vi "4 ch resonance scanner acquisition (FPGA) fixed pix clock.vi"() -> ()   [LabVIEW 2012]
uses:
  <vilib>/eio/EIONode/EIONode.xnode
  <vilib>/rvi/eio/common/nirviEmuTemplateMethod_errors.vi
  <vilib>/rvi/DataTransferAndStorage/Container/XNode/niFpgaContainer.xnode
  <vilib>/rvi/interface/RandomDataEmulation/nirviRandomDataFpgaReadWriteTemplate.vi
  <vilib>/platform/TimedLoop/XDataNode/XDataNode.xnode
  <vilib>/Platform/TimedLoop/XDataNode/nitl_modes.ctl
  <vilib>/Platform/TimedLoop/XDataNode/XDNodeRunTimeDep.lvlib
  <vilib>/Platform/TimedLoop/XDataNode/wakeup.ctl
  <vilib>/Platform/TimedLoop/XDataNode/timing_clust.ctl
panel:
  in  "lines at once":i16=4999
  in  "dwell time in ticks":i32
  in  "samples per half period":i16=4999
  in  "Start Delay (Ticks)":i16 caption="Start delay (Ticks)"
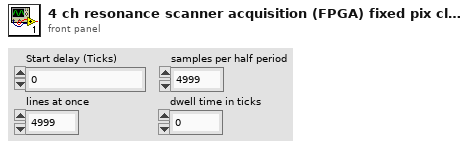
[diagram p1: front panel]
types:
  T1 = cluster{"IO Module\\AI A0":i32, "IO Module\\AI A1":i32, "IO Module\\AI A1 2":i32, "IO Module\\AI A1 3":i32}
  T2 = typedef "XDNodeRunTimeDep.lvlib/timing_clust.ctl" = cluster{"Expected End [f-1]":u64, "Actual End [f-1]":u64, "Finished Late? [f-1]":bool, "Expected End [i-1]":u64, "Actual End [i-1]":u64, "Finished Late? [i-1]":bool, "Expected Start [i]":u64, "Actual Start [i]":u64, "Expected Start [f]":u64, "Actual Start [f]":u64, "Source Name":string, "Structure Name":string, "Period":i64, "Deadline":i64, "Offset":i64, "Start":i64, "Priority":i32, "Timeout":i32, "Mode":T3, "Wakeup Reason":T4, "Error":errorcluster, "Source Type":string, "Secondary Source Type":string, "Global End Time":u64, "Global Start Time":u64, "Frame Duration":u64, "Iteration Duration":u64, "Assigned CPU":i32, "I/O Scan Engine Mode":u32}
  T3 = typedef "XDNodeRunTimeDep.lvlib/nitl_modes.ctl" = enum32{"No Change", "Process missed periods, maintain original phase", "Discard missed periods, maintain original phase", "Process missed periods, ignore original phase", "Discard missed periods, ignore original phase"}
  T4 = typedef "XDNodeRunTimeDep.lvlib/wakeup.ctl" = enum32{"Normal", "Aborted", "Asynchronous wakeup", "Timing source error", "Timed loop error", "Timeout"}
  T5 = cluster{"IO Module\\AI A0":void, "IO Module\\AI A1":void, "IO Module\\AI A2":void, "IO Module\\AI A3":void}
  T6 = cluster{"IO Module\\AI A0":i32, "IO Module\\AI A1":i32, "IO Module\\AI A2":i32, "IO Module\\AI A3":i32}
  T7 = cluster{"IO Module\\AI A0":i32, "IO Module\\AI A1":i32, i32, i32}
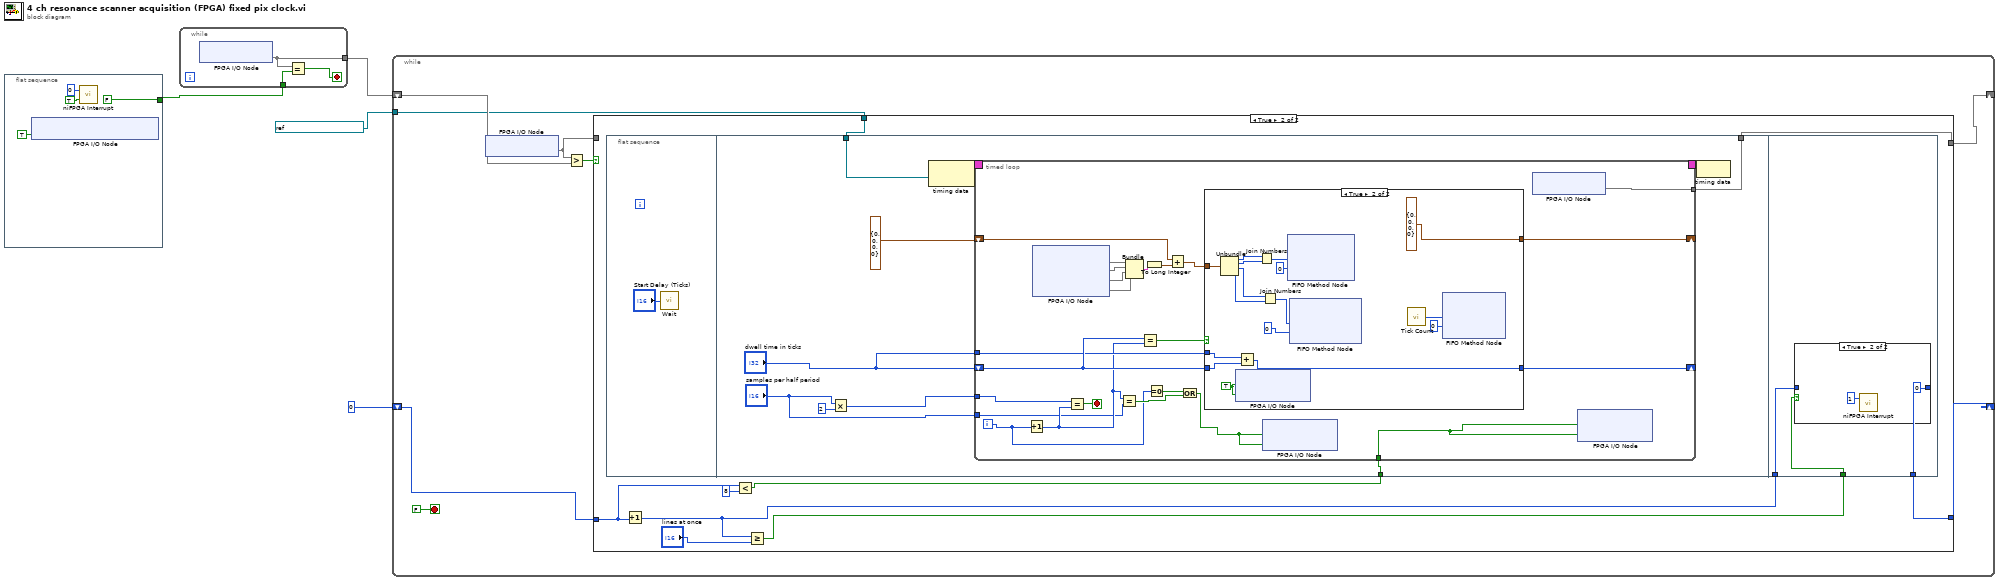
[diagram p0: block diagram]
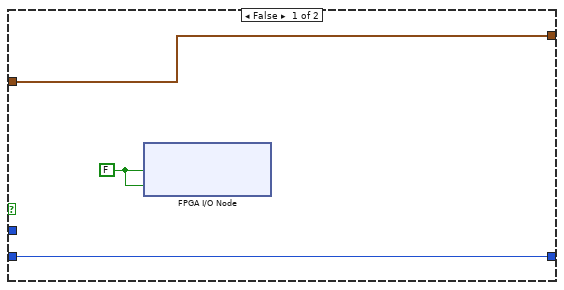
[diagram p3: hidden frame]
diagram:
  n1 = flat-sequence {
    tunnel: [FALSE ("IO Module\\DI 0")] -> w2
    frame #0 {
      n2 = xnode "FPGA I/O Node"("IO Module\\Digital Output Enable"=TRUE ("IO Module\\Digital Output Enable")) -> ()  [unwired: 1 in, 1 out]
      n3 = call <vilib>:"niFPGA Interrupt.vi"("Wait Until Cleared (F)"=TRUE, "IRQ Number (0)"=u8 0) -> ()  [unwired: 1 in]
    }
  }
  n4 = while {
    tunnel: w2 -> [w11]
    tunnel: [w9] -> w1
    stop <- w10 stop-if-true
    n5 = xnode "FPGA I/O Node"() -> ("IO Module\\DI 0"=w9)  [unwired: 1 in, 1 out]
    n6 = Equal?(x=w9, y=w11) -> (x = y?=w10:bool)
  }
  n7 = while {
    shift-right: [w18] -> _
    shift-left: w1 -> [w19]
    shift-right: [w16] -> _
    shift-left: i16 0 ("IRQ Number (0)") -> [w15]
    tunnel: refnum<k21> "40 MHz Onboard Clock" ("Source Name") -> [w13]
    stop <- FALSE stop-if-true
    n8 = xnode "FPGA I/O Node"() -> ("IO Module\\DI 0"=w12)  [unwired: 1 in, 1 out]
    n9 = Greater?(x=w12, y=w19) -> (0:w14:bool)
    n10 = case shown="True" w14 {
      tunnel: [w20 w22] -> w18
      tunnel: w15 -> [w21 w24]
      tunnel: [w21 w28] -> w16
      tunnel: w13 -> [_ w27]
      tunnel: w12 -> [w20 _]
      frame False {
      }
      frame True {
        n11 = flat-sequence {
          tunnel: w27 -> [w37]
          tunnel: w26 -> [w33]
          tunnel: [w32] -> w22
          tunnel: w30 -> [w92]
          tunnel: w29 -> [w91]
          tunnel: [w90] -> w28
          frame #0 {
            n12 = call "Wait"("Count(Ticks)"="Start Delay (Ticks)") -> ()  [unwired: 1 out]
          }
          frame #1 {
            n13 = Multiply(x="samples per half period", y=i16 2) -> (x*y=w35:i16)
            n14 = node-c288(w37) -> (w39:T2)
            n15 = timed-loop {
              tunnel: w35 -> [w63]
              shift-right: [w54] -> _
              shift-left: T1 {"IO Module\\AI A0"=0, "IO Module\\AI A1"=0, "IO Module\\AI A1 2"=0, "IO Module\\AI A1 3"=0} ("x+y") -> [w59]
              shift-right: [w57] -> _
              shift-left: "dwell time in ticks" -> [w53]
              tunnel: "dwell time in ticks" -> [w52]
              timing: w39 -> [_]
              timing-out: [_] -> w38
              tunnel: "samples per half period" -> [w43]
              tunnel: w33 -> [w49]
              tunnel: [w42] -> w32
              i -> [w45]
              stop <- w64 stop-if-true
              n16 = Increment(x=w45) -> (x+1=w44:i32)
              n17 = xnode "FPGA I/O Node"() -> ("IO Module\\AI A0"=w62, "IO Module\\AI A1"=w61, "IO Module\\AI A2"=w51, "IO Module\\AI A3"=w50)  [unwired: 4 in, 4 out]
              n18 = Equal?(x=w63, y=w44) -> (x = y?=w64:bool)
              n19 = Equal?(x=w44, y=w43) -> (x = y?=w47:bool)
              n20 = Bundle("IO Module\\AI A0"=w62, "IO Module\\AI A1"=w61, "IO Module\\AI A2"=w51, "IO Module\\AI A3"=w50) -> (w55:T5)  [unwired: 1 in]
              n21 = Equal?(x=w53, y=w44) -> (x = y?=w56:bool)
              n22 = To Long Integer(number=w55) -> (32bit integer=w60:T6)
              n23 = Equal To 0?(x=w45) -> (x = 0?=w48:bool)
              n24 = Add(x=w59, y=w60) -> (x+y=w58:T7)
              n25 = Or(x=w48, y=w47) -> (x .or. y?=w46:bool)
              n26 = case shown="True" w56 {
                tunnel: w58 -> [w67 w81]
                tunnel: [w67 T1 {"IO Module\\AI A0"=0, "IO Module\\AI A1"=0, "IO Module\\AI A1 2"=0, "IO Module\\AI A1 3"=0} ("x+y")] -> w54
                tunnel: [w66 w74] -> w57
                tunnel: w53 -> [w66 w75]
                tunnel: w52 -> [_ w76]
                frame False {
                  w65 = FALSE ("IO Module\\D0 0")
                  n27 = xnode "FPGA I/O Node"("IO Module\\D0 0"=w65, "PXI_Trig0"=w65) -> ()  [unwired: 2 in, 2 out]
                }
                frame True {
                  w68 = TRUE ("IO Module\\D0 0")
                  n28 = Unbundle(w81) -> ("IO Module\\AI A0"=w80:i32, "IO Module\\AI A1"=w79:i32, w72:i32, w71:i32)
                  n29 = xnode "FPGA I/O Node"("IO Module\\D0 0"=w68, "PXI_Trig0"=w68) -> ()  [unwired: 2 in, 2 out]
                  n30 = Add(x=w76, y=w75) -> (x+y=w74:i32)
                  n31 = Join Numbers(hi=w80, lo=w79) -> ((hi.lo)=w83:u64)
                  n32 = Join Numbers(hi=w72, lo=w71) -> ((hi.lo)=w69:u64)
                  n33 = xnode ("FIFO Method Node")("Element"=w83, "Timeout"=0) -> ()  [unwired: 1 in, 2 out]
                  n34 = xnode ("FIFO Method Node")("Element"=w69, "Timeout"=0) -> ()  [unwired: 1 in, 2 out]
                  n35 = call "Tick Count"() -> ("Tick Count(Ticks)"=w77:u32)
                  n36 = xnode ("FIFO Method Node")("Element"=w77, "Timeout"=0) -> ()  [unwired: 1 in, 2 out]
                }
              }
              n37 = xnode "FPGA I/O Node"("IO Module\\D0 1"=w46, "PXI_Trig1"=w46) -> ()  [unwired: 2 in, 2 out]
              n38 = xnode "FPGA I/O Node"() -> ("IO Module\\DI 0"=w42)  [unwired: 1 in, 1 out]
              n39 = xnode "FPGA I/O Node"("PXI_Trig2"=w49, "IO Module\\D0 2"=w49) -> ()  [unwired: 2 in, 2 out]
            }
            n40 = node-c288(w38) -> ()
          }
          frame #2 {
            n41 = case shown="True" w91 {
              tunnel: w92 -> [w93 _]
              tunnel: [w93 u8 0] -> w90
              frame False {
              }
              frame True {
                n42 = call <vilib>:"niFPGA Interrupt.vi"("IRQ Number (0)"=u8 1) -> ()  [unwired: 2 in]
              }
            }
          }
        }
        n43 = Increment(x=w24) -> (x+1=w30:i16)
        n44 = Less?(x=w24, y=i16 8) -> (x < y?=w26:bool)
        n45 = Greater Or Equal?(x=w30, y="lines at once") -> (x >= y?=w29:bool)
      }
    }
  }
